vi "Initial State Example - One-shot.vi"() -> ()   [LabVIEW 2013]
panel:
  out "Value":dbl format="%#_2g"
  in  "stop":bool
  out "Error out":errorcluster
  in  "Stream Key":string="temperature"
  in  "error in (no error)":errorcluster
  in  "Bucket Key":string="FakeSHRkyOEAP"
  in  "Access Key":string="FakeFakeVj0GLMeSHRkyOEAPFGhzWEmw"
  # "This example is meant to work with a bucket already created in Initial State. It shows that once a bucket is created, you can stream to that bucket from anywhere in your system with this single VI. To use this example, create a bucket in Initial State, place the bucket key in the field along with your access key. Hit Run. NOTE: if you forget to create the bucket first, don't worry, you can still create a bucket with the same key and your data will be there."
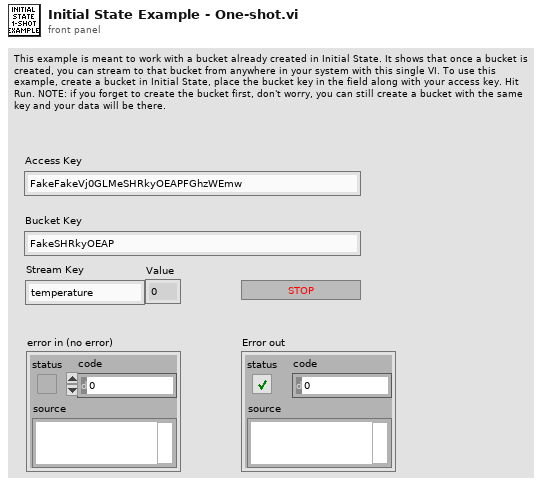
[diagram p1: front panel]
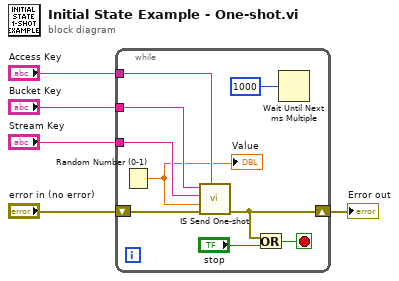
[diagram p0: block diagram]
diagram:
  n1 = while {
    tunnel: "Access Key" -> [w14]
    tunnel: "Bucket Key" -> [w12]
    tunnel: "Stream Key" -> [w11]
    shift-right: [w7] -> w3
    shift-left: "error in (no error)" -> [w13]
    stop <- w8 stop-if-true
    n2 = Random Number (0-1)() -> (number: 0 to 1=w10:dbl)
    "Value" <- w10
    n3 = call "IS Send One-shot.vi"("Access Key"=w14, "error in (no error)"=w13, "Numeric"=w10, "Stream Key"=w11, "Bucket Key"=w12) -> ("error out"=w7:errorcluster)  [unwired: 6 in]
    n4 = Or(x=w7, y="stop") -> (x .or. y?=w8:bool)
    n5 = Wait Until Next ms Multiple(millisecond multiple=u32 1000) -> ()  [unwired: 1 out]
  }
  "Error out" <- w3
